vi "Blend.vi"(7 "Source Name in":string, 8 "error in (no error)":errorcluster, 9 "Source Enqueuer":refnum<class "Message Enqueuer.lvclass">, 10 "Sample to Blend in":refnum<class "Sample.lvclass">, 11 "Transfer Line in":refnum<class "Transfer Line.lvclass">) -> (0 "error out":errorcluster, 2 "Source Name":string, 3 "Transfer Line out":refnum<class "Transfer Line.lvclass">)   [LabVIEW 2015, in "cRIO-Carbondioxide.lvlib" / "CO2-Actor.lvlib" / "Transfer Line.lvclass"]
uses:
  Transfer Line.lvclass
  subs/Sample/Sample.lvclass
  <vilib>/ActorFramework/Message Enqueuer/Message Enqueuer.lvclass
  Transfer Line.lvclass/Transfer Line.ctl
  subs/Sample/Read Sample From Container.vi
  CO2 Actor/CO2 Actor.lvclass
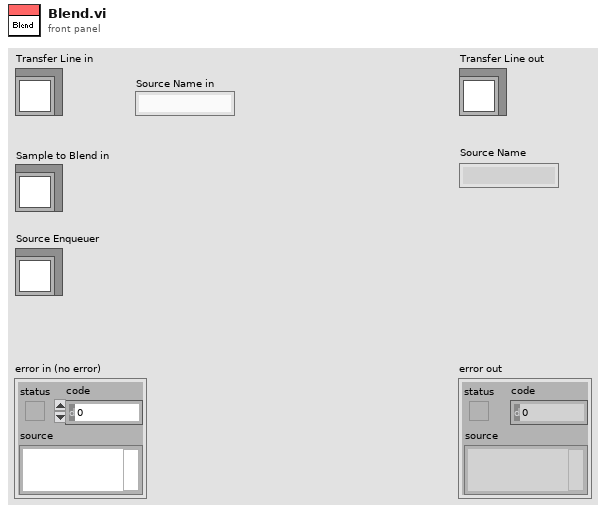
[diagram p1: front panel]
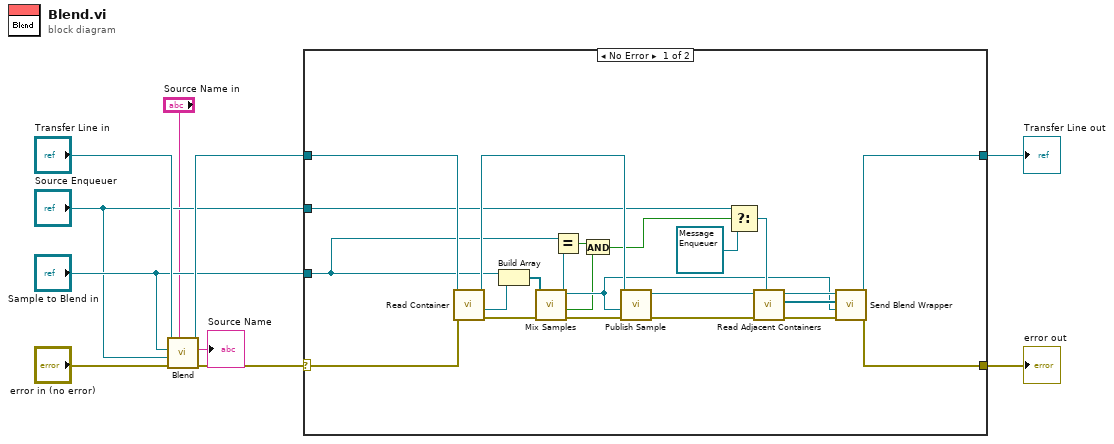
[diagram p0: block diagram]
diagram:
  n1 = call-parent "Blend.vi"("Source Name in"="Source Name in", "error in (no error)"="error in (no error)", "Source Enqueuer"="Source Enqueuer", "Sample to Blend in"="Sample to Blend in", "CO2 Actor in"="Transfer Line in") -> ("error out"=w9:errorcluster, "Source Name"=→"Source Name":string, "CO2 Actor out"=w7:refnum<class "Transfer Line.lvclass">)  [unwired: 4 in]
  n2 = case shown="No Error" w9 {
    selector: w9 -> [w31 w34]
    tunnel: [w16 w34] -> w4
    tunnel: [w26 w33] -> w3
    tunnel: w7 -> [w32 w33]
    tunnel: "Sample to Blend in" -> [w13 _]
    tunnel: "Source Enqueuer" -> [w19 _]
    frame No Error {
      n3 = call "Read Container.vi"("error in (no error)"=w31, "Transfer Line in"=w32) -> ("error out"=w30:errorcluster, "Sample"=w29:refnum<class "Sample.lvclass">, "Transfer Line out"=w27:refnum<class "Transfer Line.lvclass">)  [unwired: 5 in, 2 out]
      n4 = Build Array(w13, w29) -> (w23:refnum<class "Sample.lvclass">[])
      n5 = call "Mix Samples.vi"("error in (no error)"=w30, "Samples In"=w23) -> ("error out"=w28:errorcluster, "is clean?"=w12:bool, "Sample out"=w14:refnum<class "Sample.lvclass">)  [unwired: 6 in, 1 out]
      n6 = Equal?(x=w13, y=w14) -> (x = y?=w15:bool)
      n7 = And(x=w15, y=w12) -> (x .and. y?=w11:bool)
      n8 = call-dynamic "Publish Sample.vi"("error in (no error)"=w28, "Sample in"=w14, "Transfer Line in"=w27) -> ("error out"=w24:errorcluster, "Transfer Line out"=w25:refnum<class "Transfer Line.lvclass">)  [unwired: 7 in]
      n9 = Select(t=w19, s=w11, f=refnum<class "Message Enqueuer.lvclass"> refnum ("Source Enqueuer")) -> (s? t:f=w18:refnum<class "Message Enqueuer.lvclass">)
      n10 = call "Read Adjacent Containers.vi"("Exclude Source"=w18, "error in (no error)"=w24, "Transfer Line in"=w25) -> ("error out"=w22:errorcluster, "Adjacent Containers"=w21:refnum<class "Message Enqueuer.lvclass">[], "Transfer Line out"=w20:refnum<class "Transfer Line.lvclass">)  [unwired: 6 in]
      n11 = call-dynamic "Send Blend Wrapper.vi"("error in (no error)"=w22, "Sample to Blend"=w14, "Send to"=w21, "CO2 Actor in"=w20) -> ("error out"=w16:errorcluster, "CO2 Actor out"=w26:refnum<class "Transfer Line.lvclass">)  [unwired: 6 in]
    }
    frame Error {
    }
  }
  "error out" <- w4
  "Transfer Line out" <- w3
